vi "Init String on Multiple Controls.vi"(11 "Controls":refnum<vi>[](array[refnum]) caption="컨트롤") -> ()   [LabVIEW 2018, in "Library-Ctrl.lvlib"]
uses:
  Library-Ctrl.lvlib
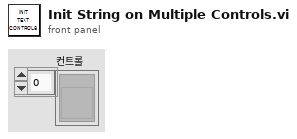
[diagram p1: front panel]
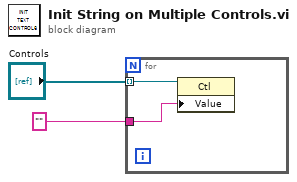
[diagram p0: block diagram]
diagram:
  n1 = for {
    tunnel: "Controls" -> [w4] mode=indexing
    tunnel: "" -> [w3]
    n2 = property class="Ctl"(reference=w4, "Value"=w3) -> ()  [unwired: 1 in, 2 out]
  }
